vi "Open Event Arguments.vi"(8 "error in":errorcluster, 11 "VI Refnum":refnum<vi>) -> (0 "error out":errorcluster)   [LabVIEW 2019, in "Panther Dashboard.lvlib"]
uses:
  Panther Dashboard.lvlib
  <vilib>/Utility/traverseref.llb/TRef TravTarget.ctl
  <vilib>/Utility/traverseref.llb/VI Scripting - Traverse.lvlib
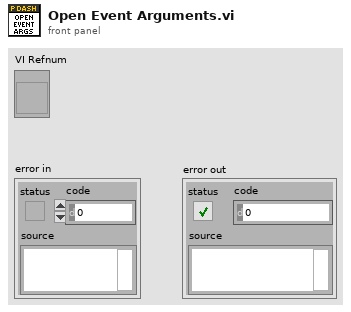
[diagram p1: front panel]
types:
  T1 = typedef "TRef TravTarget.ctl" = enum16{"FP", "BD", "Other"}
  T2 = enum32{"not a typedef", "typedef", "strict typedef", "class private data"}
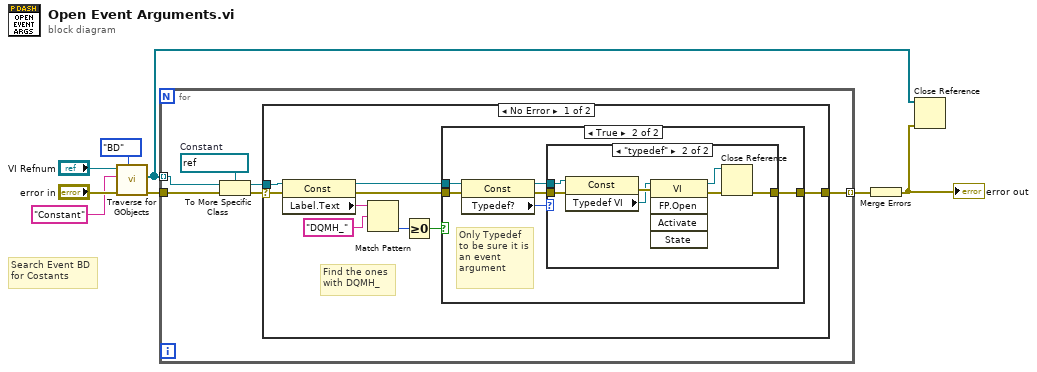
[diagram p0: block diagram]
diagram:
  # "Search Event BD\nfor Costants"
  n1 = call <vilib>:"Traverse for GObjects.vi"("Traverse Target"=TRef_TravTarget."BD", "error in (no error)"="error in", "Class Name"="Constant", "VI Refnum"="VI Refnum") -> ("error out"=w7:errorcluster, "References"=w3:refnum<vi>[])  [unwired: 4 in, 2 out]
  n2 = for {
    tunnel: w3 -> [w9] mode=indexing
    tunnel: [w13] -> w2 mode=indexing
    tunnel: w7 -> [w12]
    w10 = refnum<vi> refnum  # Constant
    n3 = To More Specific Class(target class=w10, reference=w9, error in=w12) -> (specific class reference=w11:refnum<vi>, error out=w14:errorcluster)
    n4 = case shown="No Error" w14 {
      selector: w14 -> [w23 w39]
      tunnel: w11 -> [w20 _]
      tunnel: [w21 w39] -> w13
      frame No Error {
        # "Find the ones\nwith DQMH_"
        n5 = property class="Const"(reference=w20, error in=w23) -> (reference out=w15:refnum<vi>, error out=w22:errorcluster, "Label.Text"=w19:string)
        n6 = Match Pattern(string=w19, regular expression="DQMH_") -> (offset past match=w17:i32)  [unwired: 1 in, 3 out]
        n7 = Greater Or Equal To 0?(x=w17) -> (x >= 0?=w16:bool)
        n8 = case shown="True" w16 {
          tunnel: w15 -> [_ w27]
          tunnel: w22 -> [w24 w30]
          tunnel: [w24 w28] -> w21
          frame False {
          }
          frame True {
            # "Only Typedef\nto be sure it is\nan event\nargument"
            n9 = property class="Const"(reference=w27, error in=w30) -> (reference out=w25:refnum<vi>, error out=w29:errorcluster, "Typedef?"=w26:T2)
            n10 = case shown="\"typedef\"" w26 {
              tunnel: w25 -> [_ w34]
              tunnel: [w31 w35] -> w28
              tunnel: w29 -> [w31 w36]
              frame Default {
              }
              frame "typedef" {
                n11 = property class="Const"(reference=w34, error in=w36) -> (error out=w37:errorcluster, "Typedef VI"=w33:refnum<vi>)  [unwired: 1 out]
                n12 = invoke class="VI" method="FP.Open"(reference=w33, error in=w37) -> (reference out=w32:refnum<vi>, error out=w38:errorcluster)  [unwired: 3 in, 3 out]
                n13 = Close Reference(reference=w32, error in (no error)=w38) -> (error out=w35:errorcluster)
              }
            }
          }
        }
      }
      frame Error {
      }
    }
  }
  n14 = Merge Errors(w2) -> (w6:errorcluster)
  "error out" <- w6
  n15 = Close Reference(reference=w3, error in (no error)=w6) -> ()  [unwired: 1 out]
